vi "New PDF.vi"(0 "PDF Path":path, 1 "Overwrite?":bool, 2 "Captions":cluster{"Image":T2, "Table":T2, "Font":T3}={"Image"={"Caption"="", "Separator"="", "Position"=enum."Above"}, "Table"={"Caption"="", "Separator"="", "Position"=enum."Above"}, "Font"={"Name"="", "Size"=-1.0, "Color"=0, "Style"={"Bold"=FALSE, "Italic"=FALSE, "Underline"=FALSE, "Strikeout"=FALSE}}}, 5 "Page Setup":T23={"Page Size"=1, "Orientation"=enum."Portrait", "Custom Layout"={"Width"=216.0, "Height"=279.0}, "Margins"={"Left"=25.0, "Right"=25.0, "Top"=25.0, "Bottom"=25.0}} {"Page Size" items=["Custom", "LETTER", "NOTE", "LEGAL", "TABLOID", "EXECUTIVE", "POSTCARD", "A0", "A1", "A2", "A3", "A4", "A5", "A6", "A7", "A8", "A9", "A10", "B0", "B1", "B2", "B3", "B4", "B5", "B6", "B7", "B8", "B9", "B10", "ARCH_E", "ARCH_D", "ARCH_C", "ARCH_B", "ARCH_A", "FLSA", "FLSE", "HALFLETTER", "_11X17", "ID_1", "ID_2", "ID_3", "LEDGER", "CROWN_QUARTO", "LARGE_CROWN_QUARTO", "DEMY_QUARTO", "ROYAL_QUARTO", "CROWN_OCTAVO", "LARGE_CROWN_OCTAVO", "DEMY_OCTAVO", "ROYAL_OCTAVO", "SMALL_PAPERBACK", "PENGUIN_SMALL_PAPERBACK", "PENGUIN_LARGE_PAPERBACK"]}, 9 "PDF Details":T9={"Title"="", "Subject"="", "Keywords"="", "Author"="", "Creator"="Exaprom PDF"}, 11 "Unit (default = mm)":T1=enum."mm", 12 "Default Font":T3={"Name"="Helvetica", "Size"=12.0, "Color"=0, "Style"={"Bold"=FALSE, "Italic"=FALSE, "Underline"=FALSE, "Strikeout"=FALSE}}, 14 "Default Paragraph":T6={" Aligment"=enum."JUSTIFY", "Line spacing"=enum."1.0"}) -> (4 "PDF Report":T22(xcontrol), 15 "error out":errorcluster)   [LabVIEW 2012]
doc: "Set the default values:\n1) Captions;\n2) Overwrite?;\n3) File or Directory path;\n4) Page Setup;\n5) PDF Details;\n6) Unit (default mm);\n7) Default font;\n8) Default Paragraph;\n\n<B>1) Captions </B>\nCaptions for tables and figures.\n\n<B>2) Overwrite?</B>\n\n<B>3) File or Directory path</B>\n\n<B>4)Page Setup</B>\n- Page size\n- Orientation\n- Margins\n- Custom layout (if Page size = custom)\n\n<B>5) PDF Details</B> \n- Title\n- Subject\n- Keyword\n- Author\n- Creator\n\n<B>6) Unit (default mm)</B>\nmm or in: unit used in all the report except when the unit \"point\" is specified\n\n<B>7) Default font</B>\n\nDefault font for all the report (fonts available in C:\\Windows\\Fonts).\n\n<B>8) Default Paragraph</B>\n- Alignment\n- Line Spacing\n\n<B>FRANÇAIS </B>\n\nCréation du rapport avec les paramètres par défauts:\n\n1) Légendes \"Captions\";\n2) Écrire par dessus un fichier existant \"Overwrite?\"\n3) Répertoire ou le nom du fichier \"File or Directory path\";\n4) Format des pages \"Page Setup\";\n5) Détails du fichier PDF \"PDF Details\";\n6) Unité par défaut \"Unit (default mm)\";\n7) Police de caractères par défaut \"Default font\";\n8) Interligne et l'alignement par défaut \"Default Paragraph\";\n\n<B>1) Légendes \"Captions\"</B>\nLes intitulés génériques pour les légendes (Captions) des figures et tableaux.\n\n<B>2) Écrire par dessus un fichier existant \"Overwrite?\"</B>\n\n<B>3) Répertoire ou le nom du fichier \"File or Directory path\";</B>\nLe répertoire ou le nom du fichier (chemin complet) à utiliser.\n\n<B>4) Format des pages \"Page Setup\" </B>\nFormat des pages incluant:\n- l'orientation (portrait ou paysage)\n- les marges;\n- la taille exacte si c'est un format personnalisé.\n\n<B>5) Détails du fichier PDF \"PDF Details\"</B> (métadonnées)\n- titre\n- sujet\n- mots-clés\n- auteur\n- créateur\n\n<B>6) Unité par défaut \"Unit (default mm)\"</B>\nmm or in: l'unité utilise dans l'ensemble du rapport excepté ou l'unité \"point\" spécifiée.\n\n<B>7) Police de caractères par défaut \"Default font\"</B>\n\nPolice de caractères par défaut du rapport (police disponible dans C:\\Windows\\Fonts).\n\n<B>8) Interligne et l'alignement par défaut \"Default Paragraph\"</B>\n- alignement;\n- interligne (1.0, 1.5 et 2.0)\n\nVersion 1.0\nDeveloped by Jean-Marc Simard\nCopyright © 2010, Exaprom Inc.\nAll rights reserved.\nLicense: BSD\n\nWith iTextSharp 4.1.6 (http://itextsharp.sourceforge.net)\nunder Mozilla Public License Version 1.1\n(http://www.mozilla.org/MPL/MPL-1.1.html)"
uses:
  Controls/Page setup.ctl
  Controls/Page size.ctl
  Controls/Page Orientation.ctl
  Controls/Page Layout Custom.ctl
  Controls/Page margins.ctl
  Controls/PDF Report Xcontrol/PDF Report.xctl
  Controls/PDF Details.ctl
  Controls/Font cluster.ctl
  Controls/Font size.ctl
  Controls/Font color.ctl
  Controls/Paragraphe cluster.ctl
  Controls/Texte alignement.ctl
  Controls/Line spacing.ctl
  Controls/Image or Table Caption.ctl
  Controls/Unit.ctl
  C:/Users/MaxCorp/Documents/TopPerm - Base/DLL/itextsharp.dll
  DLL/itextsharp.dll
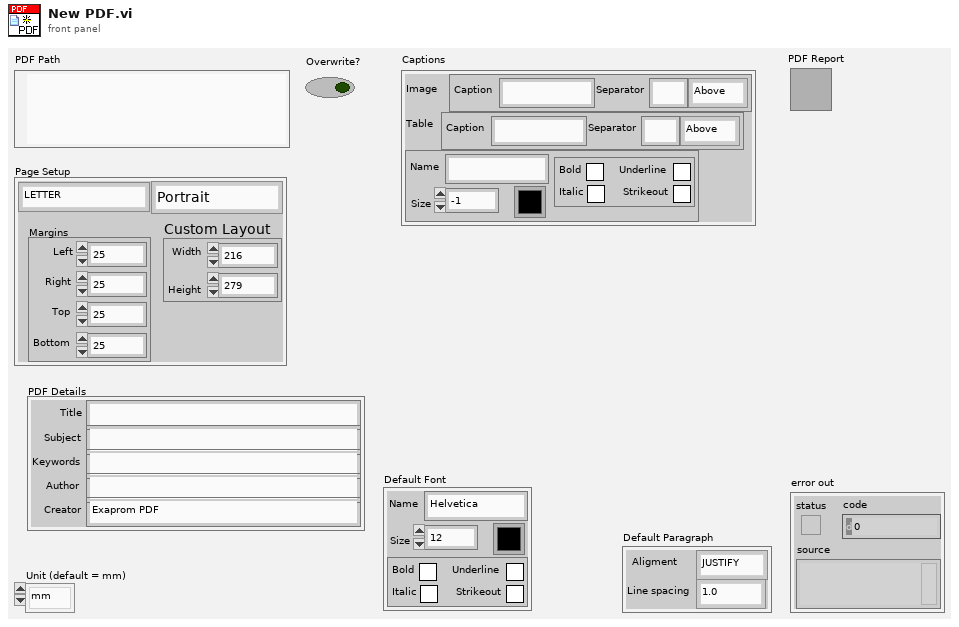
[diagram p1: front panel]
types:
  T1 = typedef "Unit.ctl" = enum16{"inch", "mm"}
  T2 = typedef "Image or Table Caption.ctl" = cluster{"Caption":string, "Separator":string, "Position":enum16{"Above", "Below"}}
  T3 = typedef "Font cluster.ctl" = cluster{"Name":string, "Size":T4, "Color":T5, "Style":cluster{"Bold":bool, "Italic":bool, "Underline":bool, "Strikeout":bool}}
  T4 = typedef "Font size.ctl" = sgl
  T5 = typedef "Font color.ctl" = u32
  T6 = typedef "Paragraphe cluster.ctl" = cluster{" Aligment":T7, "Line spacing":T8}
  T7 = typedef "Texte alignement.ctl" = enum16{"Select", "CENTER", "JUSTIFY", "LEFT", "RIGHT"}
  T8 = typedef "Line spacing.ctl" = enum16{"Select", "1.0", "1.5", "2.0"}
  T9 = typedef "PDF Details.ctl" = cluster{"Title":string, "Subject":string, "Keywords":string, "Author":string, "Creator":string}
  T10 = typedef "Page dimensions.ctl" = cluster{"Start at page":i32, "Orientation":T11, "widht":sgl, "height":sgl, "Margin left":sgl, "Margin right":sgl, "Margin top":sgl, "Margin bottom":sgl}
  T11 = typedef "Page Orientation.ctl" = enum16{"Portrait", "Landscape"}
  T12 = typedef "Header Footer [ ].ctl" = T13[]
  T13 = typedef "Header Footer cluster.ctl" = cluster{"Start page":i32, "Type":T14, "Alignment":T15, "Vertical Alignement":T16, "Image (%)":sgl, "Page #":T17, "Text":string, "Path":string, "Font":T3, "Font refnum":refnum<k24>, "Line":cluster{"Line":T18, "Thickness (points)":sgl, "Colour":T5}}
  T14 = typedef "Header Footer Type.ctl" = enum16{"Select", "Text", "Text + hyperlink", "Page number", "Image", "Image + hyperlink"}
  T15 = typedef "Header footer horiz alignment.ctl" = enum16{"Left", "Center", "Right"}
  T16 = typedef "Cell Vertical alignment.ctl" = enum16{"TOP", "MIDDLE", "BOTTOM"}
  T17 = typedef "Page number.ctl" = cluster{"Text 1":string, "Text 2":string, "Text 3":string}
  T18 = typedef "Header Footer Line.ctl" = enum16{"No line", "Horizontal line"}
  T19 = typedef "Watermark cluster2.ctl" = cluster{"Show? (F)":bool, "Type":enum16{"Image", "Text"}, "Opacity (%)":sgl, "Rotate(°)":sgl, "Position":cluster{"Position":T20, "X":sgl, "Y":sgl}, "Image path":path, "Scaled(%)":sgl, "Image refnum":refnum<k24>, "Text":string, "Font":cluster{"Name":string, "Size":T4, "Color":T5}, "Font refnum":refnum<k24>, "Alignment":T15, "Automatic":bool}
  T20 = typedef "Watermark Position.ctl" = enum16{"Absolute", "Center (page)", "Center (text section)"}
  T21 = typedef "System Fonts.ctl" = cluster{"Font name [ ]":string[], "Font and file names [ ]":cluster{"Font name":string, "File name":string}[]}
  T22 = cluster{"Document":refnum<k24>, "Writer":refnum<k24>, "Default Font":refnum<k24>, "Default Font cluster":T3, "Path":path, "Unit (default = mm)":T1, "Paragraphe cluster":T6, "Pages dimensions [ ]":T10[], "Captions":cluster{"Image":T2, "Image counter":u16, "Table":T2, "Table counter":u16, "Font":T3}, "Header":T12, "Footer":T12, "Watermark ":T19, "Actual VI name":string, "System Fonts":T21}
  T23 = typedef "Page setup.ctl" = cluster{"Page Size":T24, "Orientation":T11, "Custom Layout":T25, "Margins":T26}
  T24 = typedef "Page size.ctl" = i32
  T25 = typedef "Page Layout Custom.ctl" = cluster{"Width":sgl, "Height":sgl}
  T26 = typedef "Page margins.ctl" = cluster{"Left":sgl, "Right":sgl, "Top":sgl, "Bottom":sgl}
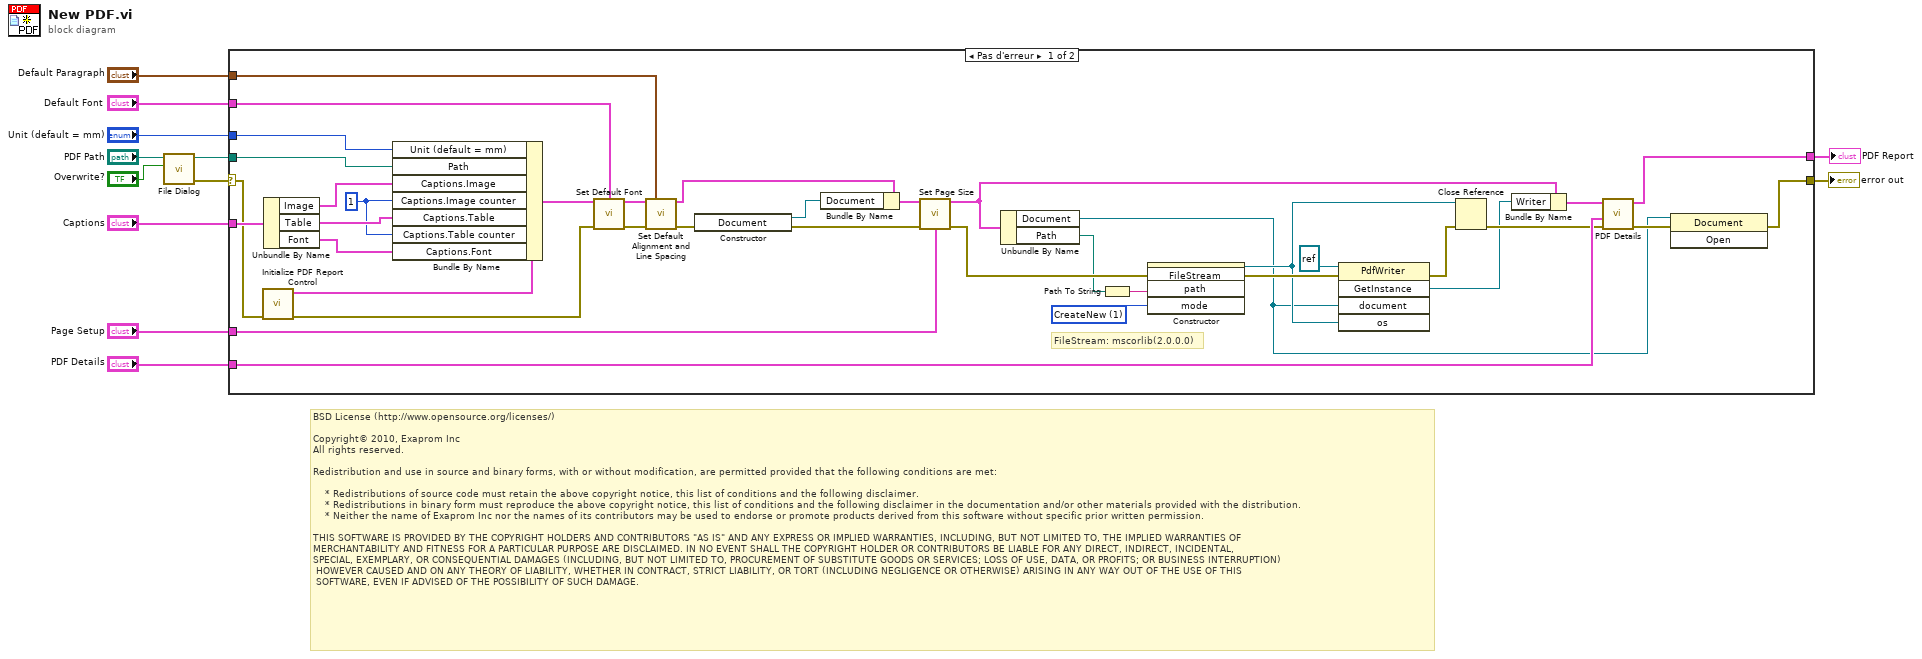
[diagram p0: block diagram]
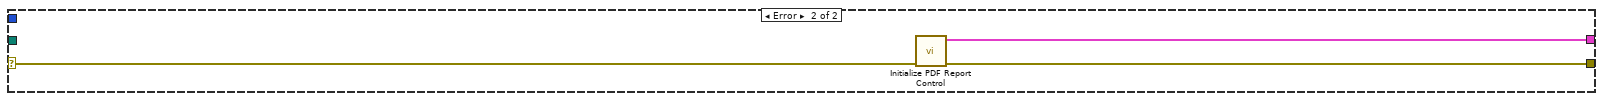
[diagram p2: hidden frame]
diagram:
  # "BSD License (http://www.opensource.org/licenses/)\n\nCopyright© 2010, Exaprom Inc\nAll rights reserved.\n\nRedistribution and use in source and binary forms, with or without modification, are permitted provided that the following conditions are met:\n\n    * Redistributions of source code must retain the above copyright notice, this list of conditions and the following disclaimer.\n    * Redistributions in binary form must reproduce the above copyright notice, this list of conditions and the following disclaimer in the documentation and/or other materials provided with the distribution.\n    * Neither the name of Exaprom Inc nor the names of its contributors may be used to endorse or promote products derived from this software without specific prior written permission.\n\nTHIS SOFTWARE IS PROVIDED BY THE COPYRIGHT HOLDERS AND CONTRIBUTORS \"AS IS\" AND ANY EXPRESS OR IMPLIED WARRANTIES, INCLUDING, BUT NOT LIMITED TO, THE IMPLIED WARRANTIES OF \nMERCHANTABILITY AND FITNESS FOR A PARTICULAR PURPOSE ARE DISCLAIMED. IN NO EVENT SHALL THE COPYRIGHT HOLDER OR CONTRIBUTORS BE LIABLE FOR ANY DIRECT, INDIRECT, INCIDENTAL,\nSPECIAL, EXEMPLARY, OR CONSEQUENTIAL DAMAGES (INCLUDING, BUT NOT LIMITED TO, PROCUREMENT OF SUBSTITUTE GOODS OR SERVICES; LOSS OF USE, DATA, OR PROFITS; OR BUSINESS INTERRUPTION)\n HOWEVER CAUSED AND ON ANY THEORY OF LIABILITY, WHETHER IN CONTRACT, STRICT LIABILITY, OR TORT (INCLUDING NEGLIGENCE OR OTHERWISE) ARISING IN ANY WAY OUT OF THE USE OF THIS\n SOFTWARE, EVEN IF ADVISED OF THE POSSIBILITY OF SUCH DAMAGE."
  n1 = call "File Dialog.vi"("Overwrite?"="Overwrite?", "Path In"="PDF Path") -> ("error out"=w6:errorcluster, "Path Out"=w8:path)  [unwired: 1 in, 7 out]
  n2 = case shown="Pas d'erreur" w6 {
    selector: w6 -> [w14 w52]
    tunnel: "Page Setup" -> [w50 _]
    tunnel: "PDF Details" -> [w49 _]
    tunnel: "Default Font" -> [w22 _]
    tunnel: "Default Paragraph" -> [w29 _]
    tunnel: w8 -> [w35 _]
    tunnel: [w17 w53] -> w5
    tunnel: "Captions" -> [w37 _]
    tunnel: "Unit (default = mm)" -> [w20 _]
    tunnel: [w15 w51] -> w1
    frame No Error {
      w26 = u16 1 ("Captions.Image counter")
      w45 = 1 items=["CreateNew"=1, "Create"=2, "Open"=3, "OpenOrCreate"=4, "Truncate"=5, "Append"=6] ("mode")
      # "FileStream: mscorlib(2.0.0.0)"
      n3 = call "Initialize PDF Report Control .vi"("error in (no error)"=w14) -> ("error out (no error)"=w25:errorcluster, "PDF Report"=w33:T22)  [unwired: 9 out]
      n4 = Unbundle By Name(w37) -> ("Image"=w39:T2, "Table"=w38:T2, "Font"=w40:T3)
      n5 = Bundle By Name(cluster=w33, "Unit (default = mm)"=w20, "Path"=w35, "Captions.Image"=w39, "Captions.Image counter"=w26, "Captions.Table"=w38, "Captions.Table counter"=w26, "Captions.Font"=w40) -> (w27:T22)
      n6 = call "Set Default Font.vi"("Document Ref IN"=w27, "Font"=w22, "error in (no error)"=w25) -> ("Document Ref OUT"=w28:T22, "error out"=w24:errorcluster)  [unwired: 11 out]
      n7 = call "Set Default Alignment and Line Spacing.vi"("PDF Report IN"=w28, "Default Paragraph"=w29, "error in (no error)"=w24) -> ("PDF Report IN"=w21:T22, "error out"=w23:errorcluster)  [unwired: 11 out]
      n8 = constructor class="Document"(error in=w23) -> (reference out=w30:refnum<k24>, error out=w32:errorcluster)  [unwired: 2 in, 1 out]
      n9 = Bundle By Name(cluster=w21, "Document"=w30) -> (w31:T22)
      n10 = call "Set Page Size.vi"("PDF Report IN"=w31, "Page setup"=w50, "error in (no error)"=w32) -> ("PDF Report OUT"=w36:T22, "error OUT"=w44:errorcluster)  [unwired: 11 out]
      n11 = Unbundle By Name(w36) -> ("Document"=w16:refnum<k24>, "Path"=w34:path)
      n12 = Path To String(path=w34) -> (string=w46:string)
      n13 = constructor class="FileStream" ("Constructor Node")(error in=w44, "path"=w46, "mode"=w45) -> (reference out=w42:refnum<k24>, error out=w47:errorcluster)  [unwired: 2 in, 3 out]
      n14 = invoke class="PdfWriter" method="GetInstance"(reference=refnum<k24> refnum, error in=w47, "document"=w16, "os"=w42) -> (error out=w43:errorcluster, "GetInstance"=w13:refnum<k24>)  [unwired: 1 in, 3 out]
      n15 = Close Reference(reference=w42, error in (no error)=w43) -> (error out=w19:errorcluster)
      n16 = Bundle By Name(cluster=w36, "Writer"=w13) -> (w41:T22)
      n17 = call "PDF Details.vi"("error in (no error)"=w19, "PDF Details"=w49, "PDF Report IN"=w41) -> ("error out"=w18:errorcluster, "PDF Report OUT"=w15:T22)  [unwired: 7 out]
      n18 = invoke class="Document" method="Open"(reference=w16, error in=w18) -> (error out=w17:errorcluster)  [unwired: 1 in, 2 out]
    }
    frame Error {
      n19 = call "Initialize PDF Report Control .vi"("error in (no error)"=w52) -> ("error out (no error)"=w53:errorcluster, "PDF Report"=w51:T22)  [unwired: 9 out]
    }
  }
  "error out" <- w5
  "PDF Report" <- w1
